vi "QI_GrabImage.vi"(8 "error in (no error)":errorcluster, 9 "Image Width":u32, 10 "Image Height":u32, 11 "Camera Handle":u32) -> (0 "error out":errorcluster, 1 "GrabImage err":u32, 2 "data":u16[][](array[numeric]), 3 "Camera Handle":u32)   [LabVIEW 2013]
uses:
  Debug/QImaging.dll
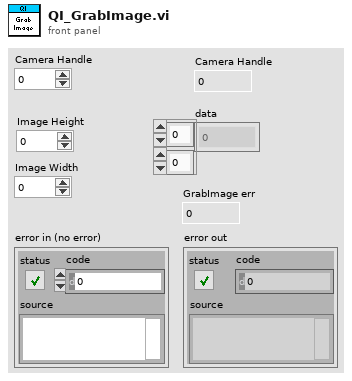
[diagram p1: front panel]
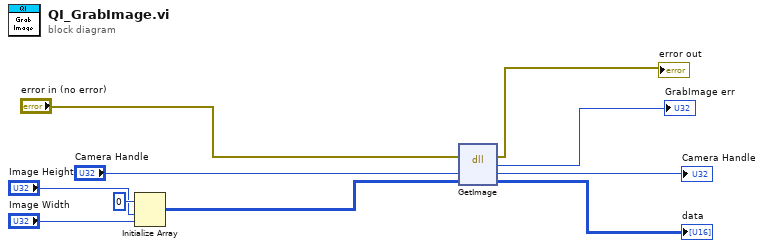
[diagram p0: block diagram]
diagram:
  n1 = Initialize Array(u16 0 ("element"), "Image Height", "Image Width") -> (w1:u16[][])
  n2 = dll-call lib="C:/Users/vernier/Documents/Visual Studio 2012/Projects/QImaging/Debug/QImaging.dll" fn="GetImage"(error in="error in (no error)", "handle"="Camera Handle", "data"=w1) -> (error out=→"error out":errorcluster, "return type"=→"GrabImage err":u32, "handle"=→"Camera Handle":u32, "data"=→"data":u16[][])  [unwired: 2 in, 1 out]
